vi "DestroyClone.vi"(8 "error in (no error)":errorcluster, 9 "Exit via Stop Module Req?":bool, 10 "Wait for Module to stop?":bool, 11 "ModuleAdmin":refnum<class "ModuleAdmin.lvclass">) -> (0 "error out":errorcluster, 1 "External Launch":bool, 3 "Mod Admin out":refnum<class "ModuleAdmin.lvclass">)   [LabVIEW 2014, in "FgenModule.lvlib"]
uses:
  FgenModule.lvlib
  <userlib>/NIST/ModuleAdminLib/ModuleAdmin/ModuleAdmin.lvclass
  <userlib>/NIST/ModuleAdminLib/ModuleAdmin/ModuleAdmin.lvclass/ModuleAdmin.ctl
  <userlib>/NIST/ModuleAdminLib/ModuleAdmin/Accessors/Read CloneRegRef.vi
  <userlib>/NIST/ModuleAdminLib/CloneRegistration/CloneRegistration.lvclass
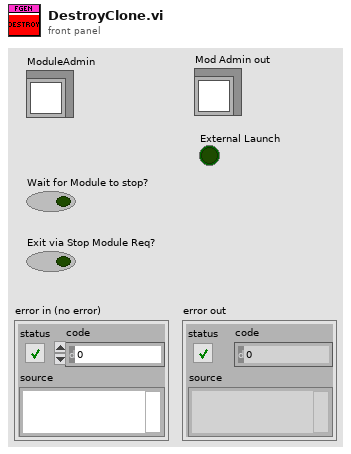
[diagram p1: front panel]
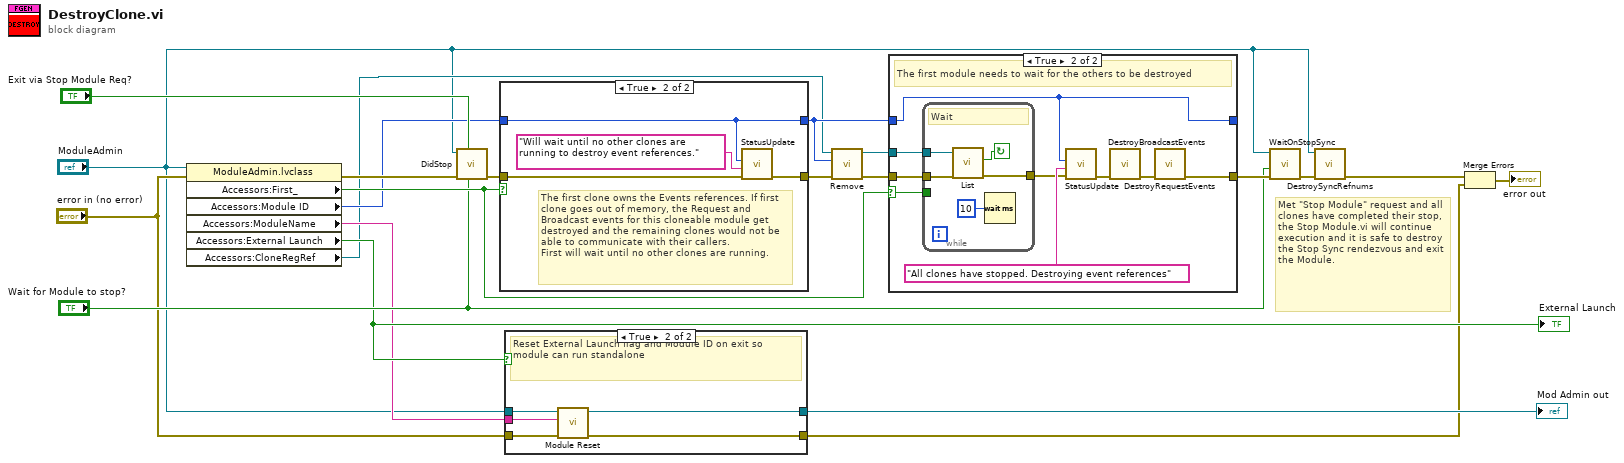
[diagram p0: block diagram]
diagram:
  # "Met \"Stop Module\" request and all clones have completed their stop, the Stop Module.vi will continue execution and it is safe to destroy the Stop Sync rendezvous and exit the Module."
  n1 = property class="ModuleAdmin.lvclass"(reference="ModuleAdmin", error in="error in (no error)") -> (error out=w21:errorcluster, "Accessors:First_"=w17:bool, "Accessors:Module ID"=w4:i32, "Accessors:ModuleName"=w8:string, "Accessors:External Launch"=w10:bool, "Accessors:CloneRegRef"=w3:refnum<data-value>)  [unwired: 1 out]
  "External Launch" <- w10
  n2 = call "DidStop.vi"("Wait for Module to stop?"="Wait for Module to stop?", "Exit via Stop Module Req?"="Exit via Stop Module Req?", "error in (no error)"=w21, "ModuleAdmin"="ModuleAdmin") -> ("error out"=w19:errorcluster)  [unwired: 7 in]
  n3 = case shown="True" w17 {
    tunnel: w19 -> [w23 w27]
    tunnel: w4 -> [w22 w24]
    tunnel: [w23 w25] -> w18
    tunnel: [w22 w24] -> w15
    frame False {
    }
    frame True {
      # "The first clone owns the Events references. If first clone goes out of memory, the Request and Broadcast events for this cloneable module get destroyed and the remaining clones would not be able to communicate with their callers.\nFirst will wait until no other clones are running."
      n4 = call "StatusUpdate.vi"("error in (no error)"=w27, "Status"="Will wait until no other clones are running to destroy event references." ("format string"), "ModuleID"=w24) -> ("error out"=w25:errorcluster)  [unwired: 8 in]
    }
  }
  n5 = case shown="True" w10 {
    tunnel: "error in (no error)" -> [w28 w34]
    tunnel: w8 -> [_ w33]
    tunnel: "ModuleAdmin" -> [w29 w32]
    tunnel: [w29 w31] -> w7
    tunnel: [w28 w30] -> w5
    frame False {
    }
    frame True {
      # "Reset External Launch flag and Module ID on exit so module can run standalone"
      n6 = call <userlib>:"Module Reset.vi"("error in (no error)"=w34, "ModuleName"=w33, "Mod Admin in"=w32) -> ("error out"=w30:errorcluster, "Mod Admin out"=w31:refnum<class "ModuleAdmin.lvclass">)  [unwired: 7 in]
    }
  }
  "Mod Admin out" <- w7
  n7 = call <userlib>:"Remove.vi"("error in (no error)"=w18, "Module ID"=w15, "CloneRegRef"=w3) -> ("error out"=w16:errorcluster, "CloneRegRef"=w2:refnum<data-value>)  [unwired: 6 in, 1 out]
  n8 = case shown="True" w17 {
    selector: w17 -> [_ w44]
    tunnel: w16 -> [w35 w45]
    tunnel: w15 -> [w36 w38]
    tunnel: [w35 w39] -> w14
    tunnel: [w36 w38] -> _
    tunnel: w2 -> [_ w37]
    frame False {
    }
    frame True {
      # "The first module needs to wait for the others to be destroyed"
      n9 = while {
        tunnel: w45 -> [w50]
        tunnel: w44 -> [_]
        tunnel: [w49] -> w42
        tunnel: w37 -> [w46]
        stop <- w48 continue-if-true
        # "Wait"
        n10 = call <userlib>:"List.vi"("error in (no error)"=w50, "CloneRegRef"=w46) -> ("error out"=w49:errorcluster, "Found?"=w48:bool)  [unwired: 4 in, 4 out]
        n11 = Wait (ms)(milliseconds to wait=u32 10) -> ()  [unwired: 1 out]
      }
      n12 = call "StatusUpdate.vi"("error in (no error)"=w42, "Status"="All clones have stopped. Destroying event references", "ModuleID"=w38) -> ("error out"=w41:errorcluster)  [unwired: 8 in]
      n13 = call "DestroyBroadcastEvents.vi"("error in (no error)"=w41) -> ("error out"=w40:errorcluster)  [unwired: 10 in]
      n14 = call "DestroyRequestEvents.vi"("error in (no error)"=w40) -> ("error out"=w39:errorcluster)  [unwired: 10 in]
    }
  }
  n15 = call <userlib>:"WaitOnStopSync.vi"("error in (no error)"=w14, "WaitForModuleToStop?"="Wait for Module to stop?", "ModuleAdmin"="ModuleAdmin") -> ("error out"=w12:errorcluster)  [unwired: 7 in, 1 out]
  n16 = call <userlib>:"DestroySyncRefnums.vi"("error in (no error)"=w12, "ModuleAdmin"="ModuleAdmin") -> ("error out"=w11:errorcluster)  [unwired: 9 in]
  n17 = Merge Errors(w11, w5) -> (→"error out":errorcluster)
